vi "Construct Multiplexed Messenger.vi"(5 "Log Alias":string, 7 "Log Instance":refnum<class "LoggerReference.lvclass">, 8 "Connections To Make":i32=-1, 9 "Port":u16, 10 "Connection State Change Callback":refnum<class "IConnectionStateChangeCallback.lvclass">, 11 "Packet Return":refnum<class "IPacket Return.lvclass">) -> (0 "error out":errorcluster, 3 "Multiplexed Messenger Out":refnum<data-value>)   [LabVIEW 2019, in "Network Messenger.lvlib" / "Multiplexed Messenger.lvclass"]
uses:
  <vilib>/gpm_packages/@cs/Network-interface/Source/Network Messenger/Multiplexed Messenger/Multiplexed Messenger.lvclass
  <vilib>/gpm_packages/@cs/Network-interface/Source/MessagingInterfaces/IConnectionStateChangeCallback/IConnectionStateChangeCallback.lvclass
  <vilib>/gpm_packages/@cs/Network-interface/Source/Network Messenger/IPacket Return/IPacket Return.lvclass
  <vilib>/gpm_packages/@cs/event-logger/Source/Composed Log/LoggerReference/LoggerReference.lvclass
  <vilib>/gpm_packages/@cs/Network-interface/Source/Network Messenger/Header Data Packet Return/Header Data Packet Return.lvclass/Header Data Packet Return.ctl
  <vilib>/gpm_packages/@cs/Network-interface/Source/Network Messenger/Write Strategy/Write Strategy.lvclass
  C:/Program Files/National Instruments/LabVIEW 2019/vi.lib/gpm_packages/@cs/Network-interface/Source/MessagingInterfaces/IWriteStrategy/IWriteStrategy.lvclass
  <vilib>/gpm_packages/@cs/Network-interface/Source/Network Messenger/ReadStrategy/ReadStrategy.lvclass
  C:/Program Files/National Instruments/LabVIEW 2019/vi.lib/gpm_packages/@cs/Network-interface/Source/MessagingInterfaces/IReadStrategy/IReadStrategy.lvclass
  <vilib>/gpm_packages/@cs/Network-interface/Source/Network Messenger/Multiplexed Messenger/Multiplexed Messenger.lvclass/Multiplexed Messenger.ctl
  <vilib>/gpm_packages/@cs/Network-interface/Source/Create Ref Message/Create Ref Message.lvclass/Create Ref Message.ctl
  <vilib>/ActorFramework/Message Enqueuer/Message Enqueuer.lvclass/Message Enqueuer.ctl
  <vilib>/ActorFramework/Message Enqueuer/Enqueue.vi
  <vilib>/gpm_packages/@cs/Network-interface/Source/MultiplexedConnectionHandler/MultiplexedConnectionHandler/MultiplexedConnectionHandler.lvclass
  C:/Program Files/National Instruments/LabVIEW 2019/vi.lib/gpm_packages/@cs/Network-interface/Source/PersistantConnectionHandler/PersistantConnectionHandler/PersistantConnectionHandler.lvclass
  C:/Program Files/National Instruments/LabVIEW 2019/vi.lib/ActorFramework/Actor/Actor.lvclass
  <vilib>/gpm_packages/@cs/Network-interface/Source/Network Messenger/Header Data Packet Return/Header Data Packet Return.lvclass
  C:/Program Files/National Instruments/LabVIEW 2019/vi.lib/gpm_packages/@cs/Network-interface/Source/MessagingInterfaces/IMessageReturnPolicy/IMessageReturnPolicy.lvclass
  <vilib>/gpm_packages/@cs/Network-interface/Source/TCP Interface/TCP Server/TCP Server.lvclass
  C:/Program Files/National Instruments/LabVIEW 2019/vi.lib/gpm_packages/@cs/Network-interface/Source/IConnectionFactory/IConnectionFactory.lvclass
  <vilib>/gpm_packages/@cs/Network-interface/Source/Create Ref Message/Create Ref Message.lvclass
  C:/Program Files/National Instruments/LabVIEW 2019/vi.lib/ActorFramework/Message/Message.lvclass
  <vilib>/ActorFramework/Message Priority Queue/Priority Enqueue.vi
  <vilib>/gpm_packages/@cs/Network-interface/Source/PersistantConnectionHandler/PersistantConnectionHandler/PersistantConnectionHandler.lvclass
  <vilib>/ActorFramework/Actor/Actor.lvclass
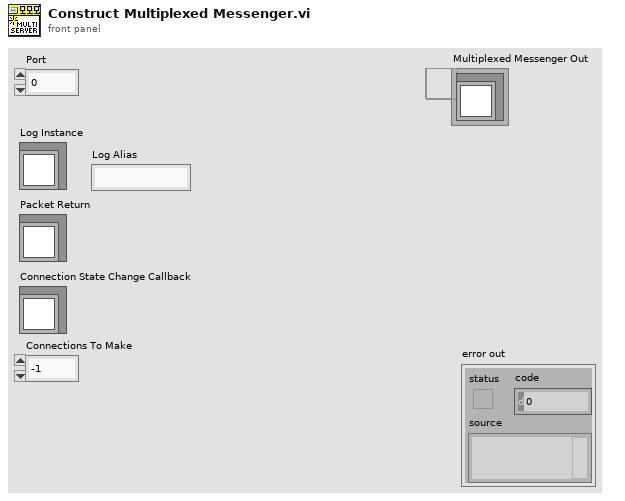
[diagram p1: front panel]
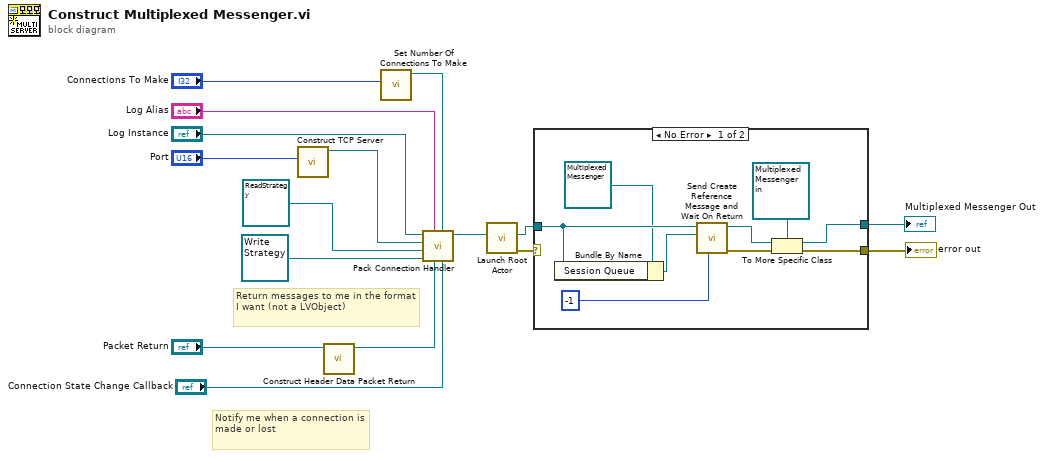
[diagram p0: block diagram]
diagram:
  # "Return messages to me in the format I want (not a LVObject)"
  # "Notify me when a connection is made or lost"
  n1 = call <vilib>:"Construct TCP Server.vi"("Port"="Port") -> ("TCP Server out"=w6:refnum<class "TCP Server.lvclass">)  [unwired: 10 in]
  n2 = call <vilib>:"Construct Header Data Packet Return.vi"("Packet Return"="Packet Return") -> ("Header Data Packet Return out"=w15:refnum<class "Header Data Packet Return.lvclass">)  [unwired: 10 in]
  n3 = call <vilib>:"Set Number Of Connections To Make.vi"("Connections To Make"="Connections To Make") -> ("MultiplexedConnectionHandler out"=w2:refnum<class "MultiplexedConnectionHandler.lvclass">)  [unwired: 9 in, 1 out]
  n4 = call <vilib>:"Pack Connection Handler.vi"("State Change Callback"="Connection State Change Callback", "PersistantConnectionHandler in"=w2, "Message Return Policy"=w15, "Log Alias"="Log Alias", "Write Strategy"=refnum<class "Write Strategy.lvclass"> refnum ("Network Messenger.lvlib:Write Strategy.lvclass"), "Read Strategy"=refnum<class "ReadStrategy.lvclass"> refnum ("Network Messenger.lvlib:ReadStrategy.lvclass"), "Connection Factory Type"=w6, "Log Instance"="Log Instance") -> ("PersistantConnectionHandler out"=w13:refnum<class "MultiplexedConnectionHandler.lvclass">)  [unwired: 3 in]
  n5 = call <vilib>:"Launch Root Actor.vi"("Actor"=w13) -> ("error out"=w12:errorcluster, "Actor's Enqueuer"=w11:refnum<class "Message Enqueuer.lvclass">)  [unwired: 9 in]
  n6 = case shown="No Error" w12 {
    selector: w12 -> [_ w26]
    tunnel: w11 -> [w24 _]
    tunnel: [w21 _] -> w3
    tunnel: [w20 w26] -> w4
    frame No Error {
      n7 = Bundle By Name(cluster=refnum<class "Multiplexed Messenger.lvclass"> refnum ("Multiplexed Messenger in"), "Session Queue"=w24) -> (w25:refnum<class "Multiplexed Messenger.lvclass">)
      n8 = call <vilib>:"Send Create Reference Message and Wait On Return.vi"("timeout in ms (-1)"=-1, "Object"=w25, "Message Enqueuer in"=w24) -> ("error out"=w23:errorcluster, "Object Reference"=w22:refnum<data-value>)  [unwired: 7 in]
      n9 = To More Specific Class(target class=refnum<data-value> refnum ("data value reference"), reference=w22, error in=w23) -> (specific class reference=w21:refnum<data-value>, error out=w20:errorcluster)
    }
    frame Error {
    }
  }
  "error out" <- w4
  "Multiplexed Messenger Out" <- w3
